vi "LS336_read_temp.vi"(6 "Data Source (0:Kelvin)":u16(ring) items=["Kelvin", "Celsius", "Sensor Units"], 9 "Serial Configuration":T1={"Baud Rate"=57600, "Parity"=1, "Data Bits"=7, "Stop Bits"=10, "Flow Control"=0} {"Flow Control" items=["None", "XON/XOFF", "RTS/CTS", "XON/XOFF & RTS/CTS", "DTR/DSR", "XON/XOFF & DTR/DSR"]; "Stop Bits" items=["1.0"=10, "1.5"=15, "2.0"=20]; "Data Bits" items=["7"=7, "8"=8]; "Parity" items=["None", "Odd", "Even", "Mark", "Space"]; "Baud Rate" items=["300"=300, "600"=600, "1200"=1200, "2400"=2400, "4800"=4800, "9600"=9600, "19200"=19200, "38400"=38400, "57600"=57600]}, 10 "Input (0:A)":u16(ring) items=["A", "B", "C", "D"], 11 "VISA Refnum in":refnum<visa-resource-name>) -> (3 "Sensor Data":dbl)   [LabVIEW 2017]
uses:
  <instrlib>/Lake Shore 336/Public/Data/Sensor Data (Single Reading).vi
  <instrlib>/Lake Shore 336/Lake Shore 336.lvlib
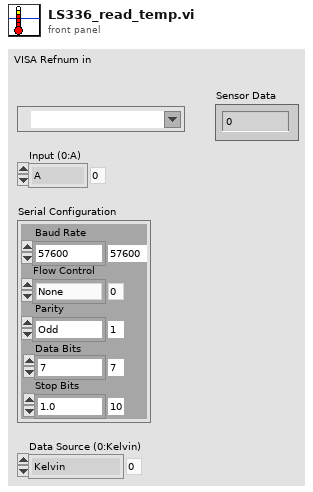
[diagram p1: front panel]
types:
  T1 = cluster{"Baud Rate":u32, "Parity":u16, "Data Bits":u16, "Stop Bits":u16, "Flow Control":u16}
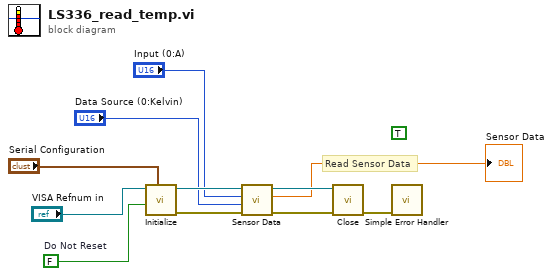
[diagram p0: block diagram]
diagram:
  (unwired) TRUE ("append to file? (new file:F)")
  w4 = FALSE  # Do Not Reset
  # "Read Sensor Data"
  n1 = call <instrlib>:"Initialize.vi"("Serial Configuration"="Serial Configuration", "Reset (True)"=w4, "VISA resource name"="VISA Refnum in") -> ("error out"=w11:errorcluster, "VISA resource name out"=w10:refnum<visa-resource-name>)  [unwired: 7 in]
  n2 = call-poly <instrlib>:"Sensor Data.vi"("error in (no error)"=w11, "Data Source (0:Kelvin)"="Data Source (0:Kelvin)", "Input (0:A)"="Input (0:A)", "VISA resource name"=w10) -> ("error out"=w9:errorcluster, "Sensor Data"=→"Sensor Data":dbl, "VISA resource name out"=w8:refnum<visa-resource-name>)  [unwired: 5 in]
  n3 = call <instrlib>:"Close.vi"("error in (no error)"=w9, "VISA resource name"=w8) -> ("error out"=w3:errorcluster)  [unwired: 9 in]
  n4 = call <vilib>:"Simple Error Handler.vi"("error in (no error)"=w3) -> ()  [unwired: 4 in, 5 out]
